vi "Set Popup Value.vi"(8 "error in (no error)":errorcluster, 11 "Popup in":refnum<class "Popup.lvclass">) -> (0 "error out":errorcluster, 3 "Popup out":refnum<class "Popup.lvclass">)   [LabVIEW 2017, in "Popup.lvclass"]
uses:
  Popup.lvclass
  Popup.lvclass/Popup.ctl
  <vilib>/Utility/Data Type/NI_Data Type.lvlib
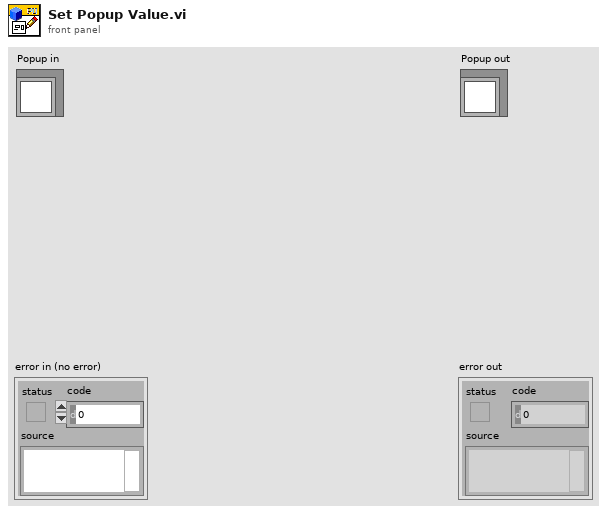
[diagram p1: front panel]
types:
  T1 = typedef "NI_Data Type.lvlib/Data Type.ctl" = enum8{"Invalid Type", "Void", "I8", "I16", "I32", "I64", "U8", "U16", "U32", "U64", "Single Float", "Double Float", "Extended Float", "Single Complex", "Double Complex", "Extended Complex", "Enum U8", "Enum U16", "Enum U32", "Enum U64", "Single Float With Unit", "Double Float With Unit", "Extended Float With Unit", "Single Complex with Unit", "Double Complex with Unit", "Extended Complex with Unit", "Boolean", "String", "Path", "Picture", "Tag", "Array", "Cluster", "Variant", "LV Variant", "Waveform", "Timestamp", "Digital Waveform", "Digital Data", "ExpressData", "Refnum", "External Data", "VI", "Poly VI", "LabVIEW Class Instance", "Fixed Point"}
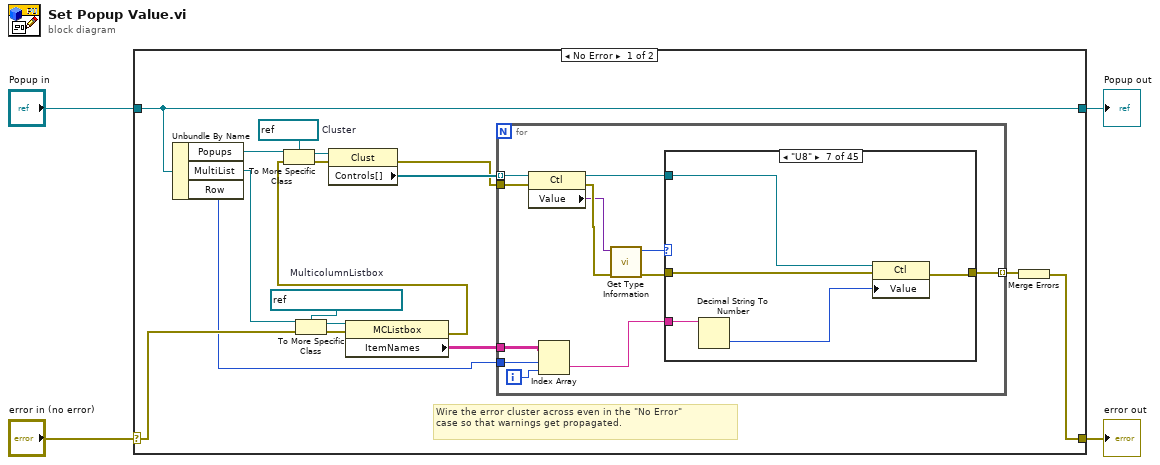
[diagram p0: block diagram]
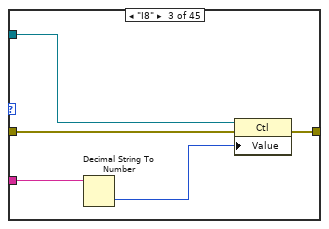
[diagram p4: hidden frame]
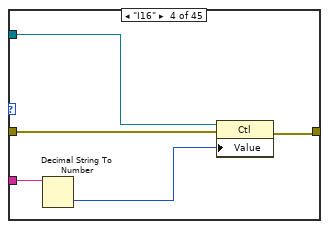
[diagram p5: hidden frame]
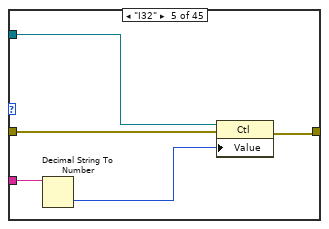
[diagram p6: hidden frame]
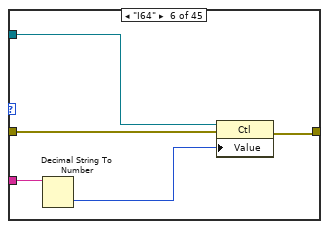
[diagram p7: hidden frame]
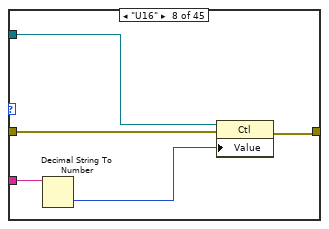
[diagram p8: hidden frame]
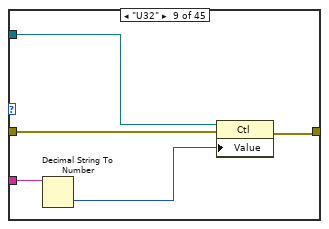
[diagram p9: hidden frame]
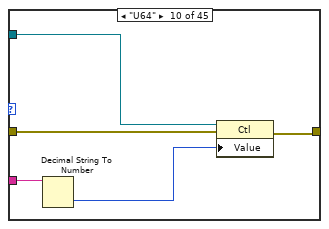
[diagram p10: hidden frame]
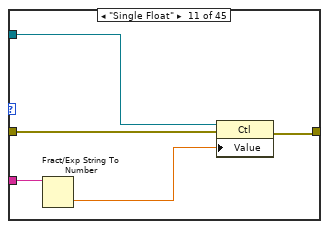
[diagram p11: hidden frame]
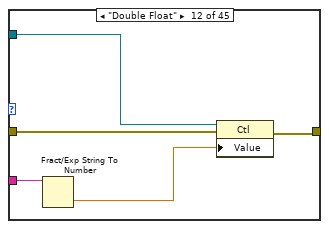
[diagram p12: hidden frame]
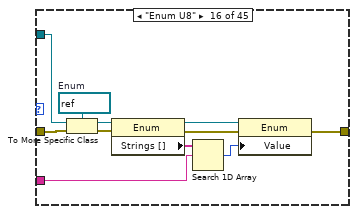
[diagram p16: hidden frame]
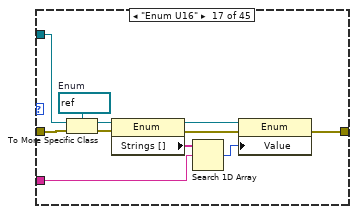
[diagram p17: hidden frame]
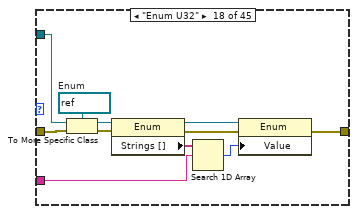
[diagram p18: hidden frame]
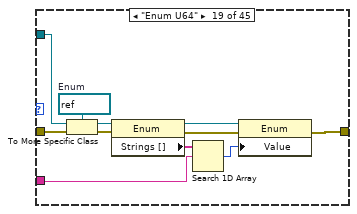
[diagram p19: hidden frame]
diagram:
  n1 = case shown="No Error" "error in (no error)" {
    selector: "error in (no error)" -> [w13 w171]
    tunnel: [w5 w171] -> w3
    tunnel: [w21 w170] -> w1
    tunnel: "Popup in" -> [w21 w170]
    frame No Error {
      w12 = refnum<vi> refnum  # MulticolumnListbox
      w19 = refnum<vi> refnum  # Cluster
      # "Wire the error cluster across even in the \"No Error\"\ncase so that warnings get propagated."
      n2 = Unbundle By Name(w21) -> ("Popups"=w20:refnum<vi>, "MultiList"=w14:refnum<vi>, "Row"=w8:u16)
      n3 = To More Specific Class(target class=w12, reference=w14, error in=w13) -> (specific class reference=w11:refnum<vi>, error out=w15:errorcluster)
      n4 = property class="MCListbox"(reference=w11, error in=w15) -> (error out=w10:errorcluster, "ItemNames"=w9:string[][])  [unwired: 1 out]
      n5 = To More Specific Class(target class=w19, reference=w20, error in=w10) -> (specific class reference=w18:refnum<vi>, error out=w17:errorcluster)
      n6 = property class="Clust"(reference=w18, error in=w17) -> (error out=w7:errorcluster, "Controls[]"=w16:refnum<vi>[])  [unwired: 1 out]
      n7 = for {
        tunnel: w16 -> [w30] mode=indexing
        tunnel: w9 -> [w33]
        tunnel: w8 -> [w31]
        tunnel: w7 -> [w29]
        tunnel: [w22] -> w6 mode=indexing
        i -> [w32]
        n8 = property class="Ctl"(reference=w30, error in=w29) -> (reference out=w24:refnum<vi>, error out=w28:errorcluster, "Value"=w25:variant)
        n9 = Index Array(array=w33, index (row)=w31, index (col)=w32) -> (element=w23:string)
        n10 = call <vilib>:"Get Type Information.vi"("error in (no error)"=w28, "Variant"=w25) -> ("error out"=w26:errorcluster, "Type"=w27:T1)  [unwired: 5 in, 3 out]
        n11 = case shown="\"U8\"" w27 {
          tunnel: w26 -> [w34 w35 w38 w45 w50 w55 w60 w65 w70 w75 w80 w85 w86 w87 w88 w94 w105 w116 w127 w133 w134 w135 w136 w137 w138 w142 w145 w151 w153 w154 w155 w156 w157 w158 w159 w160 w161 w162 w163 w164 w165 w166 w167 w168 w169]
          tunnel: [w34 w35 w39 w44 w49 w54 w59 w64 w69 w74 w79 w84 w86 w87 w88 w89 w100 w111 w122 w133 w134 w135 w136 w137 w138 w141 w146 w152 w153 w154 w155 w156 w157 w158 w159 w160 w161 w162 w163 w164 w165 w166 w167 w168 w169] -> w22
          tunnel: w24 -> [_ _ w37 w43 w48 w53 w58 w63 w68 w73 w78 w83 _ _ _ w96 w107 w118 w129 _ _ _ _ _ _ w140 w148 w150 _ _ _ _ _ _ _ _ _ _ _ _ _ _ _ _ _]
          tunnel: w23 -> [_ _ w40 w42 w47 w52 w57 w62 w67 w72 w77 w82 _ _ _ w93 w104 w115 w126 _ _ _ _ _ _ w143 w147 w149 _ _ _ _ _ _ _ _ _ _ _ _ _ _ _ _ _]
          frame "Invalid Type", Default {
          }
          frame "Void" {
          }
          frame "I8" {
            n12 = Decimal String To Number(string=w40) -> (number=w36:i32)  [unwired: 2 in, 1 out]
            n13 = property class="Ctl"(reference=w37, error in=w38, "Value"=w36) -> (error out=w39:errorcluster)  [unwired: 1 out]
          }
          frame "I16" {
            n14 = Decimal String To Number(string=w42) -> (number=w41:i32)  [unwired: 2 in, 1 out]
            n15 = property class="Ctl"(reference=w43, error in=w45, "Value"=w41) -> (error out=w44:errorcluster)  [unwired: 1 out]
          }
          frame "I32" {
            n16 = Decimal String To Number(string=w47) -> (number=w46:i32)  [unwired: 2 in, 1 out]
            n17 = property class="Ctl"(reference=w48, error in=w50, "Value"=w46) -> (error out=w49:errorcluster)  [unwired: 1 out]
          }
          frame "I64" {
            n18 = Decimal String To Number(string=w52) -> (number=w51:i32)  [unwired: 2 in, 1 out]
            n19 = property class="Ctl"(reference=w53, error in=w55, "Value"=w51) -> (error out=w54:errorcluster)  [unwired: 1 out]
          }
          frame "U8" {
            n20 = Decimal String To Number(string=w57) -> (number=w56:i32)  [unwired: 2 in, 1 out]
            n21 = property class="Ctl"(reference=w58, error in=w60, "Value"=w56) -> (error out=w59:errorcluster)  [unwired: 1 out]
          }
          frame "U16" {
            n22 = Decimal String To Number(string=w62) -> (number=w61:i32)  [unwired: 2 in, 1 out]
            n23 = property class="Ctl"(reference=w63, error in=w65, "Value"=w61) -> (error out=w64:errorcluster)  [unwired: 1 out]
          }
          frame "U32" {
            n24 = Decimal String To Number(string=w67) -> (number=w66:i32)  [unwired: 2 in, 1 out]
            n25 = property class="Ctl"(reference=w68, error in=w70, "Value"=w66) -> (error out=w69:errorcluster)  [unwired: 1 out]
          }
          frame "U64" {
            n26 = Decimal String To Number(string=w72) -> (number=w71:i32)  [unwired: 2 in, 1 out]
            n27 = property class="Ctl"(reference=w73, error in=w75, "Value"=w71) -> (error out=w74:errorcluster)  [unwired: 1 out]
          }
          frame "Single Float" {
            n28 = Fract/Exp String To Number(string=w77) -> (number=w76:dbl)  [unwired: 3 in, 1 out]
            n29 = property class="Ctl"(reference=w78, error in=w80, "Value"=w76) -> (error out=w79:errorcluster)  [unwired: 1 out]
          }
          frame "Double Float" {
            n30 = Fract/Exp String To Number(string=w82) -> (number=w81:dbl)  [unwired: 3 in, 1 out]
            n31 = property class="Ctl"(reference=w83, error in=w85, "Value"=w81) -> (error out=w84:errorcluster)  [unwired: 1 out]
          }
          frame "Single Complex" {
          }
          frame "Double Complex" {
          }
          frame "Extended Complex" {
          }
          frame "Enum U8" {
            w99 = refnum<vi> refnum  # Enum
            n32 = To More Specific Class(target class=w99, reference=w96, error in=w94) -> (specific class reference=w98:refnum<vi>, error out=w97:errorcluster)
            n33 = property class="Enum"(reference=w98, error in=w97) -> (reference out=w92:refnum<vi>, error out=w91:errorcluster, "Strings []"=w95:string[])
            n34 = Search 1D Array(1D array=w95, element=w93) -> (index of element=w90:i32)  [unwired: 1 in]
            n35 = property class="Enum"(reference=w92, error in=w91, "Value"=w90) -> (error out=w89:errorcluster)  [unwired: 1 out]
          }
          frame "Enum U16" {
            w110 = refnum<vi> refnum  # Enum
            n36 = To More Specific Class(target class=w110, reference=w107, error in=w105) -> (specific class reference=w109:refnum<vi>, error out=w108:errorcluster)
            n37 = property class="Enum"(reference=w109, error in=w108) -> (reference out=w103:refnum<vi>, error out=w102:errorcluster, "Strings []"=w106:string[])
            n38 = Search 1D Array(1D array=w106, element=w104) -> (index of element=w101:i32)  [unwired: 1 in]
            n39 = property class="Enum"(reference=w103, error in=w102, "Value"=w101) -> (error out=w100:errorcluster)  [unwired: 1 out]
          }
          frame "Enum U32" {
            w121 = refnum<vi> refnum  # Enum
            n40 = To More Specific Class(target class=w121, reference=w118, error in=w116) -> (specific class reference=w120:refnum<vi>, error out=w119:errorcluster)
            n41 = property class="Enum"(reference=w120, error in=w119) -> (reference out=w114:refnum<vi>, error out=w113:errorcluster, "Strings []"=w117:string[])
            n42 = Search 1D Array(1D array=w117, element=w115) -> (index of element=w112:i32)  [unwired: 1 in]
            n43 = property class="Enum"(reference=w114, error in=w113, "Value"=w112) -> (error out=w111:errorcluster)  [unwired: 1 out]
          }
          frame "Enum U64" {
            w132 = refnum<vi> refnum  # Enum
            n44 = To More Specific Class(target class=w132, reference=w129, error in=w127) -> (specific class reference=w131:refnum<vi>, error out=w130:errorcluster)
            n45 = property class="Enum"(reference=w131, error in=w130) -> (reference out=w125:refnum<vi>, error out=w124:errorcluster, "Strings []"=w128:string[])
            n46 = Search 1D Array(1D array=w128, element=w126) -> (index of element=w123:i32)  [unwired: 1 in]
            n47 = property class="Enum"(reference=w125, error in=w124, "Value"=w123) -> (error out=w122:errorcluster)  [unwired: 1 out]
          }
          frame "Single Float With Unit" {
          }
          frame "Double Float With Unit" {
          }
          frame "Extended Float With Unit" {
          }
          frame "Single Complex with Unit" {
          }
          frame "Double Complex with Unit" {
          }
          frame "Extended Complex with Unit" {
          }
          frame "Boolean" {
            n48 = Equal?(x="TURE", y=w143) -> (x = y?=w139:bool)
            n49 = property class="Ctl"(reference=w140, error in=w142, "Value"=w139) -> (error out=w141:errorcluster)  [unwired: 1 out]
          }
          frame "String" {
            n50 = property class="Ctl"(reference=w148, error in=w145, "Value"=w147) -> (error out=w146:errorcluster)  [unwired: 1 out]
          }
          frame "Path" {
            n51 = property class="Ctl"(reference=w150, error in=w151, "Value"=w149) -> (error out=w152:errorcluster)  [unwired: 1 out]
          }
          frame "Picture" {
          }
          frame "Tag" {
          }
          frame "Array" {
          }
          frame "Cluster" {
          }
          frame "Variant" {
          }
          frame "LV Variant" {
          }
          frame "Waveform" {
          }
          frame "Timestamp" {
          }
          frame "Digital Waveform" {
          }
          frame "Digital Data" {
          }
          frame "ExpressData" {
          }
          frame "Refnum" {
          }
          frame "External Data" {
          }
          frame "VI" {
          }
          frame "Poly VI" {
          }
          frame "LabVIEW Class Instance" {
          }
          frame "Fixed Point" {
          }
        }
      }
      n52 = Merge Errors(w6) -> (w5:errorcluster)
    }
    frame Error {
    }
  }
  "error out" <- w3
  "Popup out" <- w1
